vi "micro1.vi"(6 "flux in en entrée":string, 9 "expression régulière":string, 10 "data in":string, 11 "cmd":string) -> (3 "flux in en sortie":string)   [LabVIEW 2020]
uses:
  <vilib>/regexp/Match Regular Expression.xnode
panel:
  out "après la correspondance":string
  out "toute l'expression":string
  out "avant la correspondance":string
  # "EQISO+:HIOKI,ST5520,190416767,V2.02\\$R"
  # "EQISO+HIOKI,ST5520,AAA:EQISO-HIOKI,ST5520,BBB:EQIOCVHIOKI,BT3562CCC*$R"
  # "EQISO\\+HIOKI,ST5520,[0-9 A-Z . ,]*:EQISO\\-HIOKI,_,[0-9 A-Z . ,]*:EQIOCVHIOKI,BT3562[0-9 A-Z . , \\-]*\\$R"
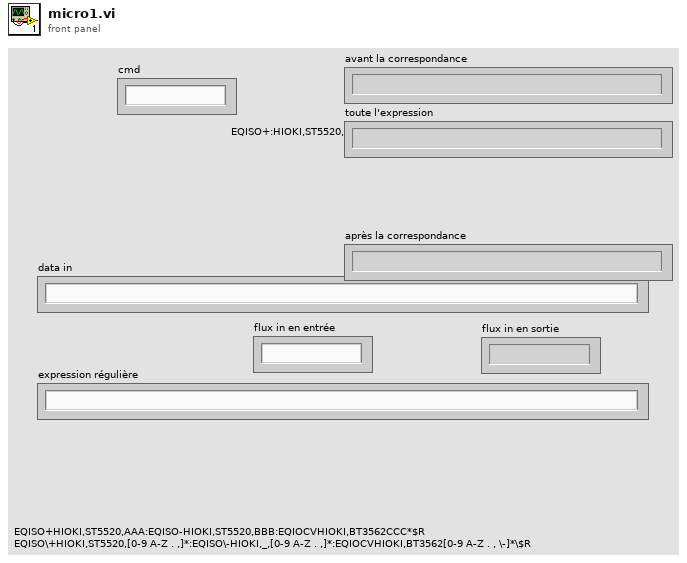
[diagram p1: front panel]
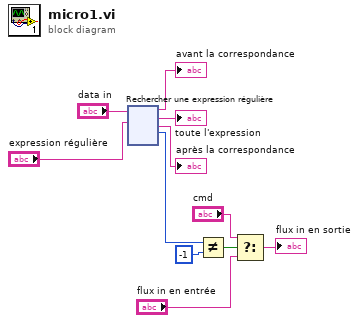
[diagram p0: block diagram]
diagram:
  n1 = xnode "Rechercher une expression régulière"("chaîne en entrée"="data in", "expression régulière"="expression régulière") -> ("avant la correspondance"=→"avant la correspondance":string, "toute l'expression"=→"toute l'expression":string, "après la correspondance"=→"après la correspondance":string, "offset après correspondance"=w6:i32)  [unwired: 4 in, 1 out]
  n2 = Not Equal? ("Différents ?")(x=w6, y=-1) -> (x != y?=w7:bool)
  n3 = Select ("Sélectionner")(t="cmd", s=w7, f="flux in en entrée") -> (s? t:f=→"flux in en sortie":string)
